vi "CreatePrivateEvents.vi"(8 "error in (no error)":errorcluster, 11 "SynchIO.USB4431":refnum<class "SynchIO.PXI-4461.lvclass">) -> (0 "error out":errorcluster, 3 "SynchIO.USB4431 out":refnum<class "SynchIO.PXI-4461.lvclass">)   [LabVIEW 2016, in "SynchIO.PXI-4461.lvclass"]
doc: "---------------------------------------------------------------\nJKI State Machine Objects™\nhttp://jki.net/state-machine-objects/\nCopyright (C) 2005-2015, JKI <info@jki.net>\nALL RIGHTS RESERVEDJKI State Machine Objects (SMO) 1.0.0.4\nJKI - JKI\nCopyright (c) 2015, JKI"
uses:
  SynchIO.PXI-4461.lvclass
  SynchIO.PXI-4461.lvclass/SynchIO.PXI-4461.ctl
  Typedefs/PrivateEvents--SynchIO.USB4431.Initialize.ctl
  Typedefs/PrivateEvents--SynchIO.USB4431.Init.ctl
  Typedefs/PrivateEvents--SynchIO.USB4431.Init-Event.ctl
  SynchIO/SynchIO.lvclass
panel:
  # "For instructions on how to use the JKI State Machine Objects, examples and video tutorials, visit:\nhttp://jki.net/state-machine-objects/\n\nJKI State Machine Objects™\nhttp://jki.net/state-machine-objects/\nCopyright (C) 2005-2015, JKI <info@jki.net>\nALL RIGHTS RESERVED"
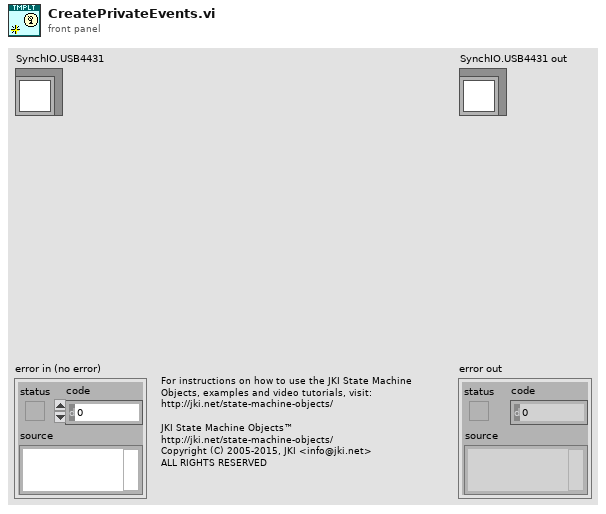
[diagram p1: front panel]
types:
  T1 = typedef "SynchIO.PXI-4461.lvclass/PrivateData--Ref.ctl" = refnum<data-value>
  T2 = typedef "SynchIO.PXI-4461.lvclass/PrivateEvents--SynchIO.USB4431.Init-Event.ctl" = bool
  T3 = typedef "SynchIO.PXI-4461.lvclass/PrivateEvents--SynchIO.USB4431.Init.ctl" = bool
  T4 = typedef "SynchIO.PXI-4461.lvclass/PrivateEvents--SynchIO.USB4431.Initialize.ctl" = bool
  T5 = typedef "SynchIO.PXI-4461.lvclass/PrivateData--Cluster.ctl" = cluster{"Configuration":T6, "Public Events":T7, "Protected Events":T8, "Data":string, "Private Events":T9}
  T6 = typedef "SynchIO.PXI-4461.lvclass/Configuration--Cluster.ctl" = cluster{"Suffix":string}
  T7 = typedef "SynchIO.PXI-4461.lvclass/PublicEvents--Cluster.ctl" = cluster{"Data Changed":refnum<user-event>, "Initialize":refnum<user-event>}
  T8 = typedef "SynchIO.PXI-4461.lvclass/ProtectedEvents--Cluster.ctl" = cluster{"API_Template":refnum<user-event>}
  T9 = typedef "SynchIO.PXI-4461.lvclass/PrivateEvents--Cluster.ctl" = cluster{"Initialize":refnum<user-event>, "Init":refnum<user-event>, "Init-Event":refnum<user-event>}
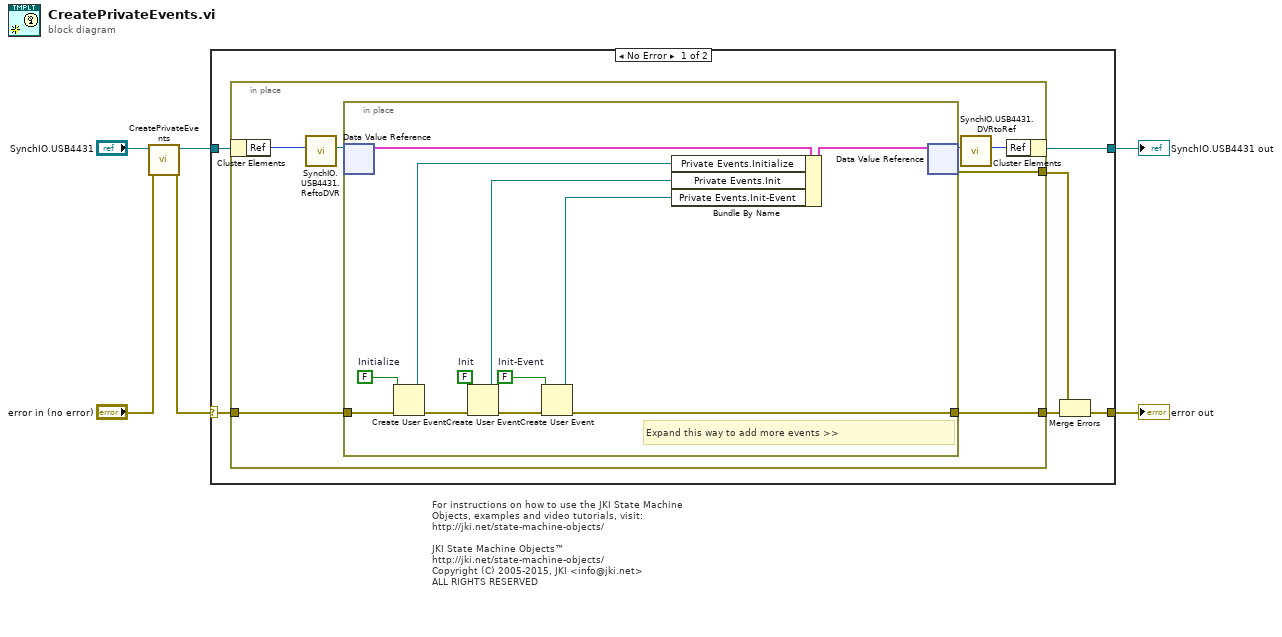
[diagram p0: block diagram]
diagram:
  # "For instructions on how to use the JKI State Machine Objects, examples and video tutorials, visit:\nhttp://jki.net/state-machine-objects/\n\nJKI State Machine Objects™\nhttp://jki.net/state-machine-objects/\nCopyright (C) 2005-2015, JKI <info@jki.net>\nALL RIGHTS RESERVED"
  n1 = call-parent "CreatePrivateEvents.vi"("error in (no error)"="error in (no error)", "SynchIO"="SynchIO.USB4431") -> ("error out"=w1:errorcluster, "SynchIO out"=w3:refnum<class "SynchIO.PXI-4461.lvclass">)  [unwired: 8 in]
  n2 = case shown="No Error" w1 {
    selector: w1 -> [w10 w33]
    tunnel: [w8 w33] -> w5
    tunnel: [w11 w32] -> w6
    tunnel: w3 -> [w12 w32]
    frame No Error {
      n3 = in-place {
        in-place-border: w10 -> [w19]
        in-place-border: [w16] -> w7
        in-place-border: [w15] -> w9
        n4 = in-place-cluster #1(w12) -> ("Ref"=w18:u32)
        n5 = call "SynchIO.USB4431.ReftoDVR.vi"("Ref"=w18) -> ("Ref"=w14:T1)  [unwired: 10 in]
        n6 = in-place {
          in-place-border: w19 -> [w31]
          in-place-border: [w22] -> w16
          w21 = T2 FALSE  # Init-Event
          w24 = T3 FALSE  # Init
          w27 = T4 FALSE  # Initialize
          # "Expand this way to add more events >>"
          n7 = in-place-dvr #2(w14) -> (w30:T5)  [unwired: 1 out]
          n8 = Create User Event(user event datatype=w27, error in=w31) -> (user event=w26:refnum<user-event>, error out=w28:errorcluster)
          n9 = Create User Event(user event datatype=w24, error in=w28) -> (user event=w23:refnum<user-event>, error out=w25:errorcluster)
          n10 = Create User Event(user event datatype=w21, error in=w25) -> (user event=w20:refnum<user-event>, error out=w22:errorcluster)
          n11 = Bundle By Name(cluster=w30, "Private Events.Initialize"=w26, "Private Events.Init"=w23, "Private Events.Init-Event"=w20) -> (w29:T5)
          n12 = in-place-dvr #2(w29) -> (w17:T1, w15:errorcluster)
        }
        n13 = call "SynchIO.USB4431.DVRtoRef.vi"("Ref"=w17) -> ("Ref"=w13:u32)  [unwired: 10 in]
        n14 = in-place-cluster #1("Ref"=w13) -> (w11:refnum<class "SynchIO.PXI-4461.lvclass">)
      }
      n15 = Merge Errors(w9, w7) -> (w8:errorcluster)
    }
    frame Error {
    }
  }
  "error out" <- w5
  "SynchIO.USB4431 out" <- w6
